vi "Get Channel Name Core.vi"(8 "error in (no error)":errorcluster, 10 "Channel Index (1)":i32=1, 11 "CS++Scope":refnum<class "CS++Scope.lvclass">) -> (0 "error out":errorcluster, 2 "Channel Name":string, 3 "CS++Scope out":refnum<class "CS++Scope.lvclass">)   [LabVIEW 2014, in "CS++Scope.lvlib" / "CS++Scope.lvclass"]
doc: "This VI returns the highest-level channel name that corresponds to the specific driver channel string that is in the channel table at an index you specify."
uses:
  CS++Scope.lvclass
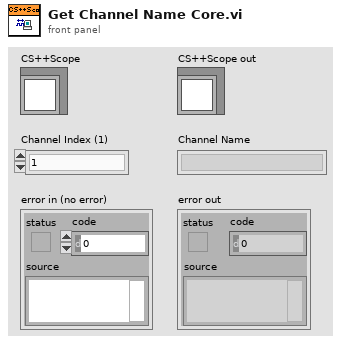
[diagram p1: front panel]
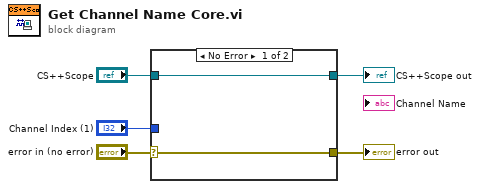
[diagram p0: block diagram]
diagram:
  n1 = case shown="No Error" "error in (no error)" {
    selector: "error in (no error)" -> [w6 w9]
    tunnel: [w6 w9] -> w4
    tunnel: [w7 w8] -> w2
    tunnel: "CS++Scope" -> [w7 w8]
    tunnel: "Channel Index (1)" -> [_ _]
    frame No Error {
    }
    frame Error {
    }
  }
  "error out" <- w4
  "CS++Scope out" <- w2
